vi "UHR-Fleezers Control (host) - 10.5.vi"() -> ()   [LabVIEW 2011]
uses:
  <vilib>/Utility/miscctls.llb/LVPoint32TypeDef.ctl
  <vilib>/Utility/miscctls.llb/LVMinMaxIncTypeDef.ctl
  <vilib>/userDefined/High Color/nirio_resource_hc.ctl
  <vilib>/Platform/TimedLoop/XDataNode/timing_clust.ctl
  <vilib>/Platform/TimedLoop/XDataNode/nitl_modes.ctl
  <vilib>/Platform/TimedLoop/XDataNode/wakeup.ctl
  <vilib>/vision/Avi1.llb/AviRefnum.ctl
  <vilib>/Instr/_visa.llb/VISA Configure Serial Port (Instr).vi
  <vilib>/FPGAPlugInAG/PCIe-7852R/niLvFpga_Open_PCIe-7852R.vi
  <vilib>/FPGAPlugInAG/PCIe-7852R/niLvFpga_Reset_PCIe-7852R.vi
  <vilib>/Utility/error.llb/Error Cluster From Error Code.vi
  <vilib>/rvi/errors/niLvFpgaAdjustHostInterfaceError.vi
  <vilib>/FPGAPlugInAG/PCIe-7852R/niLvFpga_Run_PCIe-7852R.vi
  <vilib>/express/express analysis/Spectral/Block/exnSpectralBlock spectral measurements PSD poly.vi
  <vilib>/express/express analysis/Spectral/Block/exnSpectralBlock spectral measurements PSD WFM.vi
  <vilib>/Waveform/WDTOps.llb/WDT Append Waveforms DBL.vi
  <vilib>/FPGAPlugInAG/PCIe-7852R/niLvFpga_Close_PCIe-7852R.vi
  openfpgaref.8.6.ctl
  <vilib>/Platform/TimedLoop/XDataNode/XDataNode.xnode
  <vilib>/rvi/interface/nirviOpenFPGA/nirviOpenFPGA.xnode
  FPGA Bitfiles/UHR-FleezersInst_FPGATarget_UHR-FleezersCont_AF27E570.lvbitx
  UHR-Fleezers Control (fpga) - 10.5.vi
  <vilib>/rvi/interface/nirviMethod/nirviMethod.xnode
  <vilib>/rvi/interface/nirviReadWriteControl/nirviReadWriteControl.xnode
  <vilib>/express/express analysis/Spectral/XNode/ExpressSpectralMeasurementsBlockNode.xnode
  <vilib>/rvi/interface/nirviCloseFPGA/nirviCloseFPGA.xnode
  <vilib>/Analysis/NI_AALBase.lvlib
  <vilib>/Platform/TimedLoop/XDataNode/XDNodeRunTimeDep.lvlib
  <vilib>/vision/NI_Vision_Development_Module.lvlib
  <vilib>/rvi/errors/niLvFpgaMergeErrorWithErrorCode.vi
  NiFpgaLv.dll
  <vilib>/FPGAPlugInAG/PCIe-7852R/niLvFpga_ConfigureFifo_PCIe-7852R.vi
  <vilib>/FPGAPlugInAG/PCIe-7852R/niLvFpga_ReadFifo_PCIe-7852R.vi
panel:
  out "Pump 3 cont disp":string="Left: ADig beads"
  out "Pump 1 cont disp":string="Right: DNA beads "
  in  "Ch 1 Inject Rate (ul/h)":dbl=25.0
  in  "Pump write delay (ms)":dbl=300.0
  in  "All Pump Parameters":T1={"Pump 1"={"Diameter (mm)"=4.61, "Units"=4.0, "Volume"=100.0, "Rate"=25.0}, "Pump 2"={"Diameter (mm)"=4.61, "Units"=3.0, "Volume"=0.0, "Rate"=0.0}, "Pump 3"={"Diameter (mm)"=4.61, "Units"=4.0, "Volume"=100.0, "Rate"=800.0}}
  in  "Ch 1 Inject Volume (uL)":dbl=100.0
  in  "Pump pause delay (ms)":u32
  in  "Ch 3 Inject Volume (uL)":dbl=100.0
  in  "Ch 3 Inject Rate (ul/h)":dbl=800.0
  in  "Flush Center Ch Volume (uL)":dbl=15.0
  in  "Flush Center Ch Rate (ul/m)":dbl=100.0
  in  "Inject Pump 2":bool caption="Inject Pump 2\n(Flush Center)"
  in  "Total Volume\nFlushed (uL)":dbl
  out "TTrig":cluster{dbl, dbl}(graph)
  in  "Sample Channel\nFlow":bool
  in  "Inject Pump 1":bool
  in  "Inject Pump 3":bool
  in  "Pump 1 contents":string="Bottom: DNA beads" caption="Contents"
  in  "Pump 3 contents":string="Top: ADig beads" caption="Contents"
  out "Time (s)":dbl=58.8
  in  "Index":dbl=1.0 caption="Save File Index" min=1.0 step=1.0
  in  "Scripts":T2(tab)
  in  "Fixed Traps Data\nScript":bool
  in  "Dump spot flow on?":bool=TRUE caption="Flow ON?"
  in  "Daq spot flow on":bool=TRUE caption="Flow ON?"
  in  "Cap 1 Samp Flow ON":bool=TRUE
  in  "Cap 2 Samp Flow ON":bool=TRUE
  in  "Got DNA bead":bool
  in  "Got ADig bead":bool
  in  "Cap 2 Flow ON":bool=TRUE
  in  "Cap 1 Flow ON":bool=TRUE
  in  "Cap 2 T ON":bool=TRUE
  in  "Move Cap. 2 (ADig Top)":bool
  in  "Move Cap. 1 (DNA Bottom)":bool
  in  "Cal/Data Acq. Spot":bool
  in  "Dump Beads":bool
  in  "Cap 1 T ON":bool=TRUE
  in  "Force FB Data\nScript":bool
  in  "Cap. 2 BD T1?\n(ADig T1, DNA T2)":bool
  in  "Offset 2 Set":dbl=2.0
  in  "Offset 1 Set":dbl
  in  "Cal @ (MHz)":dbl=15.25
  in  "W/ Offset 1":bool=TRUE
  in  "Offset 1 Start (MHz)":dbl=13.0
  in  "W/ Offset 2":bool
  in  "Offset 2 Start (MHz)":dbl=16.0
  in  "Cal Stage Position":i32=3
  in  "Flow ON during \nfishing?":bool=TRUE
  in  "Fish again after \nraster break?":bool=TRUE
  in  "Furthest Delta (MHz)":dbl=15.25 step=0.25
  in  "Green ON During Raster":bool
  in  "Move to Delta 2 (MHz)":dbl=13.0
  in  "Attempt Limit":dbl=15.0 caption="Limit"
  out "Attempts":dbl=15.0
  in  "Wait Before Save (s)":u32=1
  in  "Closest Delta (MHz)":dbl=9.25 step=0.25
  in  "Stop F (pN)":dbl=3.0
  in  "Then...":string(combo)="5"
  in  "Move to Delta 1 (MHz)":dbl=13.0
  in  "Tether Alarm?":bool=TRUE
  out "Tether":bool
  in  "TA Cancel Save?":bool
  in  "TA Green Off?":bool
  in  "Raster Set Upon Tether":u32=1
  in  "Save at end (5, 6)":bool
  in  "Start dipping after?":bool=TRUE
  in  "Green ON after FB ON?":bool
  in  "Remove Action Offset":bool
  in  "Stage Position To Establish FB":i32=3
  in  "Trap Trig Fl.":bool
  in  "Starting \nTrap Delta (MHz)":dbl=15.25
  in  "Trap Delta Before Moving":dbl=13.0
  in  "Wait (s)":u32=1
  in  "Green ON":bool
  in  "Start dipping after?":bool=TRUE
  in  "Fixed Traps Trap Delta (MHz)":dbl=15.25 caption="Trap Delta (MHz)"
  out "TTrig Fin Thresh (nm)":dbl
  out "TTrig Sig (nm)":dbl
  out "Threshold stored (nm)":dbl
  in  "Neg. TTrig FPGA":bool=TRUE
  in  "Test ttrig":bool
  in  "Trap Trig. (FPGA)":bool=TRUE
  out "Initializing":bool
  in  "Reinitialize":bool
  out "Triggered":bool
  out "Waiting":bool
  in  "Trap Trig. Fl.":bool
  in  "Wait to get offset (n)":u32=10
  in  "Threshold (nm)":dbl=15.0
  in  "Fl. ON time (n)":i32=90
  out "T1 x pos data":dbl[](array[numeric])=[-0.7109037245680824, -0.7109037245680824]
  out "max value":dbl=-0.9003514563721442
  out "min value":dbl=-1.184251119672945
  in  "Mean T1 Position\nto compare (nm)":dbl caption="Mean T1 for Comparison (nm)" format="%0.2f"
  out "mean":dbl=-1.0423012880225446 format="%0.2f"
  out "standard\ndeviation":dbl=0.2007473770965739 format="%0.2f"
  out "TTrig Sig (Int)":i64
  out "TTrig Fin Thresh (Int)":i64
  in  "FB Trig Integrate":u32=1
  in  "FB OFF when \nflow ON":bool
  in  "Flow ON \nduring return\nfrom dip?":bool=TRUE
  in  "Flow ON\nduring daq?":bool
  in  "Flow ON\nduring dip?":bool=TRUE
  in  "Cancel dwell":bool
  in  "Pause dwell \ntimer":bool
  in  "Dwell Duration (s)":i32=45
  in  "Green ON\nbefore dip?":bool
  in  "Cont. Repeat Dipping?":bool=TRUE
  in  "Dipping Delta (MHz)":dbl=15.0
  in  "Move trap \nbefore dip move?":bool
  in  "Save data\nafter return move?":bool
  in  "Green ON \nafter return?":bool=TRUE
  in  "Dip Trap Delta 2 (MHz)":dbl=15.0
  in  "Move trap \nafter return move?":bool
  in  "Dip Duration (s)":i32=15
  in  "Dip for Protein":bool
  in  "Dip Stage \nPosition":i32=5
  in  "Return Stage \nPosition":i32=3
  out "Dip Time (s)":i32=16
  out "Dip #":i32=5
  in  "Y change (mm)":dbl=3.0
  in  "Profile":bool
  out "Current Position":cluster{dbl, dbl, dbl}={1.5, -2.90746, -0.04434}
  in  "APD to Watch":bool
  out "Duration (s)":dbl
  in  "Action":string(combo)="Yank"
  in  "Fl. Triggered...":bool
  in  "Fl. Delta Thresh. (kHz)":dbl=0.6
  out "Waiting":bool
  out "Fl. High":bool
  in  "N pts to average":u16=6
  in  "Yank Delay (s)":dbl=3.5
  in  "Yank to Delta Array (MHz)":dbl[](array[numeric])=[16.3, 15.85, 14.85]
  in  "N Array El":u8=3 min=1 step=1
  in  "Random Choice":bool=TRUE
  in  "Force Yank":bool
  in  "Force Reset":bool
  in  "N Steps":dbl=20.0
  in  "Step Size (nm)":dbl=0.34
  in  "Save ave factor":dbl=1.0
  in  "Take Stepping Data":bool
  out "Sigma/Mean 2":dbl=0.36441577304438716 caption="Sigma/Mean" format="%#_2g"
  out "Rate sigma (Hz) 2":dbl=288.009932629414 caption="Sigma (Hz)" format="%0.2f"
  out "APD 2 Rate (Hz)":dbl=790.3333333333334 format="%#_3p"
  out "Primary Video Display":T3(plugin-control)
  out "Waveform Graph":dbl[](graph) caption="APD Line Scan"
  out "Messages":string="1:17 PM\tUHR-Fleezers ready.\r"
  in  "APD Ave N":dbl=10.0
  out "Int. Time (s)":dbl=3.0
  in  "Stop All":bool
  out "Sigma/Mean":dbl=0.18579745817752089 format="%#_2g"
  out "Rate sigma (Hz)":dbl=488.0899226323474 caption="Sigma (Hz)" format="%0.2f"
  in  "Tab Control 6":T4(tab)
  in  "APD 2 Offset":dbl
  in  "APD 1 Offset":dbl
  out "RMS (Ang)":dbl=6.074493407838442 format="%_2g"
  in  "Bead Sep. Int. Time (s)":dbl=3.0 caption="Int. Time (s)"
  in  "Below (kHz)":dbl=1.0
  in  "Above (kHz)":dbl=2.0
  in  "Adjust Scale\nto Mean":bool
  in  "Remove Offset":bool
  in  "Offset (nm)":dbl=-9.822711494362707 format="%#_3g"
  out "Mean":dbl=-2.4278133956623194 caption="Mean (pN)" format="%#_3g"
  out "Force":waveform(dbl)[](graph)=[{"t0"=timestamp(16.200000000000017 s since 1904-01-01), "dt"=0.15, "Y"=[-50.791733123427015, -51.19733990933295], "attributes"=variant("NI_ChannelName"=variant(string "T1 X"))}, {"t0"=timestamp(16.200000000000017 s since 1904-01-01), "dt"=0.15, "Y"=[45.92404992947972, 46.35376952063096], "attributes"=variant("NI_ChannelName"=variant(string "T2 X"))}]
  out "APD Chart":waveform(dbl)[](graph)=[{"t0"=timestamp(16.200000000000017 s since 1904-01-01), "dt"=0.15, "Y"=[2546.666666666667, 2813.3333333333335], "attributes"=variant("NI_ChannelName"=variant(string "APD 1"))}, {"t0"=timestamp(16.200000000000017 s since 1904-01-01), "dt"=0.15, "Y"=[720.0, 900.0], "attributes"=variant("NI_ChannelName"=variant(string "APD 2"))}]
  in  "Calibration":u16(ring)=2 items=["None", "Position", "Force"]
  out "T1 X":dbl=-50.99453651637998 caption="T1 X (pN)" format="%0.2f"
  out "T2 X":dbl=-46.13890972505534 caption="T2 X (pN)" format="%0.2f"
  out "Bead Separation":waveform(dbl)(graph)={"t0"=timestamp(16.200000000000017 s since 1904-01-01), "dt"=0.15, "Y"=[46.80967498827478, 46.86053516179577], "attributes"=variant("NI_ChannelName"=variant(string "T1 X"))}
  out "Bead Mean (nm)":dbl=47.53979851497442 caption="Mean (nm)" format="%0.2f"
  out "Difference":dbl=-97.13344624143532 caption="Difference (pN)" format="%.2g"
  in  "Take Detection Laser\nImage":bool
  out "APD 2":T3(plugin-control) caption="APD 2 (Cy5)"
  in  "Flip Green Filter":bool
  in  "Set X Only":bool
  in  "Set Y Only":bool
  out "APD 1":T3(plugin-control) caption="APD 1 (Cy3)"
  out "Detection Laser Y":T3(plugin-control)
  out "Pointer Y (V)":dbl=6.416201666310619 format="%_3g"
  out "Pointer X (V)":dbl=2.173967101046785 format="%_3g"
  in  "Set Confocal Spot (X-Y)":bool
  out "Detection Laser X":T3(plugin-control)
  out "Saved APD":dbl[][](graph)=[[2720.0, 2573.3333333333335, 2613.3333333333335, 2453.3333333333335, 2480.0, 2560.0, 2506.666666666667, 2466.666666666667, 2440.0, 2520.0, 2580.0, 2400.0, 2793.3333333333335, 2346.666666666667, 2853.3333333333335, 2453.3333333333335, 2513.3333333333335, 2713.3333333333335, 2720.0, 2633.3333333333335, 2560.0, 2693.3333333333335, 2620.0, 2613.3333333333335, 2453.3333333333335, 2566.666666666667, 2333.3333333333335, 2726.666666666667, 2806.666666666667, 2526.666666666667, 2640.0, 2606.666666666667, 2680.0, 2793.3333333333335, 2546.666666666667, 2473.3333333333335, 2593.3333333333335, 2653.3333333333335, 2566.666666666667, 2493.3333333333335, 2766.666666666667, 2446.666666666667, 2466.666666666667, 2746.666666666667, 2800.0, 2306.666666666667, 2426.666666666667, 2593.3333333333335, 2633.3333333333335, 2326.666666666667, 2693.3333333333335, 2680.0, 2726.666666666667, 2546.666666666667, 2573.3333333333335, 2446.666666666667, 2513.3333333333335, 2606.666666666667, 2686.666666666667, 2460.0, 2653.3333333333335, 2660.0, 2406.666666666667, 2706.666666666667, 2520.0, 2420.0, 2560.0, 2553.3333333333335, 2566.666666666667, 2406.666666666667, 2546.666666666667, 2433.3333333333335, 2446.666666666667, 2480.0, 2520.0, 2593.3333333333335, 2653.3333333333335, 2580.0, 2600.0, 2626.666666666667, 2686.666666666667, 2593.3333333333335, 2540.0, 2580.0, 2586.666666666667, 2626.666666666667, 2426.666666666667, 2800.0, 2693.3333333333335, 2666.666666666667, 2553.3333333333335, 2746.666666666667, 2693.3333333333335, 2880.0, 2480.0, 2540.0, 2613.3333333333335, 2573.3333333333335, 2746.666666666667, 2633.3333333333335, 3006.666666666667, 2880.0, 2813.3333333333335, 2660.0, 2653.3333333333335, 2513.3333333333335, 2526.666666666667, 2800.0, 2673.3333333333335, 2286.666666666667, 2593.3333333333335, 2260.0, 2620.0, 2653.3333333333335, 2753.3333333333335, 2413.3333333333335, 2433.3333333333335, 2506.666666666667, 2340.0, 2800.0, 2653.3333333333335, 2473.3333333333335, 2320.0, 2600.0, 2613.3333333333335, 2613.3333333333335, 2546.666666666667, 2586.666666666667, 2506.666666666667, 2860.0, 2273.3333333333335, 2540.0, 2486.666666666667, 2493.3333333333335, 2626.666666666667, 2620.0, 2466.666666666667, 2600.0, 2840.0, 2746.666666666667, 2580.0, 2760.0, 2686.666666666667, 2446.666666666667, 2600.0, 2533.3333333333335, 2800.0, 2933.3333333333335, 2580.0, 2400.0, 2540.0, 2600.0, 2580.0, 2360.0, 2480.0, 2580.0, 2486.666666666667, 2520.0, 2546.666666666667, 2626.666666666667, 2400.0, 2740.0, 2573.3333333333335, 2413.3333333333335, 2566.666666666667, 2633.3333333333335, 2500.0, 2680.0, 2393.3333333333335, 2533.3333333333335, 2633.3333333333335, 2406.666666666667, 2600.0, 2566.666666666667, 2860.0, 2713.3333333333335, 2506.666666666667, 2726.666666666667, 2560.0, 2693.3333333333335, 2633.3333333333335, 2473.3333333333335, 2593.3333333333335, 2533.3333333333335, 2533.3333333333335, 2753.3333333333335, 2440.0, 2680.0, 2593.3333333333335, 2560.0, 2440.0, 2460.0, 2506.666666666667, 2593.3333333333335, 2613.3333333333335, 2433.3333333333335, 2706.666666666667, 2666.666666666667, 2533.3333333333335, 2593.3333333333335, 2686.666666666667, 2320.0, 2553.3333333333335, 2853.3333333333335, 2686.666666666667, 2620.0, 2673.3333333333335, 2493.3333333333335, 2333.3333333333335, 2593.3333333333335, 2546.666666666667, 2553.3333333333335, 2706.666666666667, 2613.3333333333335, 2466.666666666667, 2433.3333333333335, 2633.3333333333335, 2920.0, 2480.0, 2580.0, 2346.666666666667, 2613.3333333333335, 2566.666666666667, 2626.666666666667, 2453.3333333333335, 2586.666666666667, 2700.0, 2420.0, 2520.0, 2573.3333333333335, 2626.666666666667, 2673.3333333333335, 2446.666666666667, 2526.666666666667, 2506.666666666667, 2640.0, 2500.0, 2500.0, 2473.3333333333335, 2640.0, 2500.0, 2373.3333333333335, 2706.666666666667, 2666.666666666667, 2853.3333333333335, 2460.0, 2533.3333333333335, 2706.666666666667, 2526.666666666667, 2760.0, 2506.666666666667, 2566.666666666667, 2653.3333333333335, 2646.666666666667, 2873.3333333333335, 2613.3333333333335, 2493.3333333333335, 2513.3333333333335, 2640.0, 2486.666666666667, 2740.0, 2660.0, 2653.3333333333335, 2633.3333333333335, 2906.666666666667, 2860.0, 2653.3333333333335, 2633.3333333333335, 2640.0, 2406.666666666667, 2540.0, 2613.3333333333335, 2393.3333333333335, 2506.666666666667, 2600.0, 2546.666666666667, 2653.3333333333335, 2513.3333333333335, 2633.3333333333335, 2386.666666666667, 2546.666666666667, 2893.3333333333335, 2733.3333333333335, 2593.3333333333335, 2573.3333333333335, 2580.0, 2653.3333333333335, 2666.666666666667, 2680.0, 2580.0, 2393.3333333333335, 2780.0, 2413.3333333333335, 2606.666666666667, 2600.0, 2540.0, 2546.666666666667, 2833.3333333333335, 2513.3333333333335, 2573.3333333333335, 2693.3333333333335, 2840.0, 2580.0, 2700.0, 2793.3333333333335, 2546.666666666667, 2606.666666666667, 2453.3333333333335, 2593.3333333333335, 2500.0, 2520.0, 2640.0, 2813.3333333333335, 2813.3333333333335, 2493.3333333333335, 2686.666666666667, 2673.3333333333335, 2533.3333333333335, 2480.0, 2606.666666666667, 2680.0, 2646.666666666667, 2646.666666666667, 2626.666666666667, 2433.3333333333335, 2633.3333333333335, 2540.0, 2506.666666666667, 2620.0, 2553.3333333333335, 2480.0, 2533.3333333333335, 2620.0, 2860.0, 2506.666666666667, 2753.3333333333335, 2400.0, 2493.3333333333335, 2513.3333333333335, 2713.3333333333335, 2673.3333333333335, 2473.3333333333335, 2720.0, 2580.0, 2613.3333333333335, 2533.3333333333335, 2680.0, 2413.3333333333335, 2373.3333333333335, 2566.666666666667, 2560.0, 2806.666666666667, 2633.3333333333335, 2520.0, 2526.666666666667, 2633.3333333333335, 2753.3333333333335, 2746.666666666667, 2780.0, 2780.0, 2466.666666666667, 2573.3333333333335, 2600.0, 2706.666666666667, 2506.666666666667, 2500.0, 2586.666666666667, 2646.666666666667, 2620.0, 2400.0, 2726.666666666667, 2666.666666666667, 2606.666666666667, 2553.3333333333335, 2726.666666666667, 2720.0, 2546.666666666667, 2606.666666666667, 2506.666666666667, 2573.3333333333335, 2593.3333333333335, 2660.0, 2600.0, 2580.0, 2440.0, 2846.666666666667, 2406.666666666667, 2600.0, 2573.3333333333335, 2533.3333333333335], [766.6666666666667, 786.6666666666667, 813.3333333333334, 806.6666666666667, 813.3333333333334, 813.3333333333334, 813.3333333333334, 760.0, 846.6666666666667, 873.3333333333334, 853.3333333333334, 813.3333333333334, 880.0, 853.3333333333334, 813.3333333333334, 713.3333333333334, 820.0, 826.6666666666667, 846.6666666666667, 760.0, 833.3333333333334, 733.3333333333334, 800.0, 786.6666666666667, 766.6666666666667, 760.0, 740.0, 733.3333333333334, 840.0, 773.3333333333334, 800.0, 846.6666666666667, 853.3333333333334, 913.3333333333334, 733.3333333333334, 793.3333333333334, 773.3333333333334, 793.3333333333334, 853.3333333333334, 800.0, 833.3333333333334, 893.3333333333334, 886.6666666666667, 766.6666666666667, 706.6666666666667, 813.3333333333334, 733.3333333333334, 780.0, 593.3333333333334, 846.6666666666667, 720.0, 740.0, 800.0, 726.6666666666667, 833.3333333333334, 800.0, 846.6666666666667, 740.0, 726.6666666666667, 780.0, 733.3333333333334, 706.6666666666667, 740.0, 806.6666666666667, 666.6666666666667, 980.0, 873.3333333333334, 933.3333333333334, 793.3333333333334, 913.3333333333334, 780.0, 786.6666666666667, 746.6666666666667, 846.6666666666667, 726.6666666666667, 786.6666666666667, 786.6666666666667, 686.6666666666667, 820.0, 746.6666666666667, 846.6666666666667, 720.0, 733.3333333333334, 800.0, 706.6666666666667, 766.6666666666667, 773.3333333333334, 780.0, 833.3333333333334, 853.3333333333334, 733.3333333333334, 820.0, 706.6666666666667, 673.3333333333334, 833.3333333333334, 806.6666666666667, 813.3333333333334, 700.0, 806.6666666666667, 793.3333333333334, 753.3333333333334, 886.6666666666667, 746.6666666666667, 820.0, 693.3333333333334, 720.0, 786.6666666666667, 920.0, 893.3333333333334, 760.0, 840.0, 713.3333333333334, 846.6666666666667, 793.3333333333334, 793.3333333333334, 773.3333333333334, 786.6666666666667, 813.3333333333334, 926.6666666666667, 806.6666666666667, 786.6666666666667, 820.0, 800.0, 733.3333333333334, 813.3333333333334, 826.6666666666667, 846.6666666666667, 720.0, 773.3333333333334, 760.0, 873.3333333333334, 866.6666666666667, 880.0, 766.6666666666667, 746.6666666666667, 720.0, 893.3333333333334, 793.3333333333334, 813.3333333333334, 900.0, 746.6666666666667, 866.6666666666667, 833.3333333333334, 780.0, 833.3333333333334, 733.3333333333334, 733.3333333333334, 613.3333333333334, 806.6666666666667, 880.0, 853.3333333333334, 753.3333333333334, 746.6666666666667, 893.3333333333334, 800.0, 873.3333333333334, 933.3333333333334, 733.3333333333334, 693.3333333333334, 920.0, 993.3333333333334, 720.0, 853.3333333333334, 706.6666666666667, 686.6666666666667, 793.3333333333334, 726.6666666666667, 806.6666666666667, 860.0, 813.3333333333334, 806.6666666666667, 666.6666666666667, 860.0, 793.3333333333334, 800.0, 773.3333333333334, 653.3333333333334, 853.3333333333334, 720.0, 806.6666666666667, 640.0, 993.3333333333334, 773.3333333333334, 833.3333333333334, 673.3333333333334, 786.6666666666667, 780.0, 846.6666666666667, 786.6666666666667, 866.6666666666667, 813.3333333333334, 893.3333333333334, 813.3333333333334, 746.6666666666667, 806.6666666666667, 900.0, 740.0, 813.3333333333334, 973.3333333333334, 873.3333333333334, 780.0, 720.0, 860.0, 833.3333333333334, 633.3333333333334, 746.6666666666667, 813.3333333333334, 653.3333333333334, 813.3333333333334, 940.0, 973.3333333333334, 853.3333333333334, 820.0, 773.3333333333334, 760.0, 860.0, 860.0, 733.3333333333334, 760.0, 940.0, 713.3333333333334, 713.3333333333334, 913.3333333333334, 926.6666666666667, 840.0, 766.6666666666667, 840.0, 853.3333333333334, 753.3333333333334, 746.6666666666667, 733.3333333333334, 760.0, 793.3333333333334, 780.0, 860.0, 740.0, 840.0, 853.3333333333334, 760.0, 820.0, 926.6666666666667, 566.6666666666667, 820.0, 820.0, 846.6666666666667, 846.6666666666667, 960.0, 773.3333333333334, 866.6666666666667, 746.6666666666667, 813.3333333333334, 973.3333333333334, 866.6666666666667, 686.6666666666667, 826.6666666666667, 853.3333333333334, 906.6666666666667, 866.6666666666667, 706.6666666666667, 813.3333333333334, 786.6666666666667, 800.0, 806.6666666666667, 813.3333333333334, 693.3333333333334, 886.6666666666667, 760.0, 953.3333333333334, 720.0, 873.3333333333334, 826.6666666666667, 866.6666666666667, 786.6666666666667, 733.3333333333334, 873.3333333333334, 720.0, 813.3333333333334, 780.0, 753.3333333333334, 673.3333333333334, 760.0, 833.3333333333334, 700.0, 853.3333333333334, 773.3333333333334, 926.6666666666667, 900.0, 753.3333333333334, 886.6666666666667, 820.0, 820.0, 713.3333333333334, 813.3333333333334, 720.0, 840.0, 880.0, 880.0, 773.3333333333334, 746.6666666666667, 800.0, 920.0, 900.0, 766.6666666666667, 773.3333333333334, 766.6666666666667, 800.0, 860.0, 893.3333333333334, 680.0, 780.0, 760.0, 713.3333333333334, 660.0, 806.6666666666667, 920.0, 686.6666666666667, 806.6666666666667, 793.3333333333334, 773.3333333333334, 753.3333333333334, 873.3333333333334, 753.3333333333334, 860.0, 826.6666666666667, 793.3333333333334, 833.3333333333334, 773.3333333333334, 906.6666666666667, 766.6666666666667, 813.3333333333334, 766.6666666666667, 846.6666666666667, 673.3333333333334, 826.6666666666667, 826.6666666666667, 746.6666666666667, 746.6666666666667, 873.3333333333334, 786.6666666666667, 700.0, 893.3333333333334, 786.6666666666667, 913.3333333333334, 820.0, 833.3333333333334, 820.0, 893.3333333333334, 826.6666666666667, 746.6666666666667, 760.0, 753.3333333333334, 746.6666666666667, 746.6666666666667, 893.3333333333334, 753.3333333333334, 833.3333333333334, 826.6666666666667, 880.0, 813.3333333333334, 880.0, 666.6666666666667, 806.6666666666667, 773.3333333333334, 913.3333333333334, 726.6666666666667, 793.3333333333334, 880.0, 840.0, 833.3333333333334, 866.6666666666667, 946.6666666666667, 813.3333333333334, 846.6666666666667, 826.6666666666667, 813.3333333333334, 766.6666666666667, 766.6666666666667, 720.0, 746.6666666666667, 786.6666666666667, 820.0, 846.6666666666667, 853.3333333333334, 786.6666666666667, 800.0, 820.0, 746.6666666666667, 720.0, 840.0, 806.6666666666667]] caption="Most Recent Time Trace"
  out "Trap Delta Graph":dbl[](graph)=[47.20544674943777, 46.38357473836321, 45.83818091067762, 46.35063870780333, 46.57328126817542, 46.26983509094593, 46.207785466693664, 46.12090860203374, 46.75480485600748, 45.89837089817051, 46.52249402855391, 46.74710833092389, 46.48685302300156, 45.980928940659666, 46.08378499907887, 46.29776150204533, 46.52270355958599, 45.13312371565935, 45.45279739842816, 46.12725237006576, 45.934373783395515, 46.11062060160292, 45.819898737241985, 46.427428605258385, 46.4251508638754, 46.259210180234035, 46.536328123957716, 45.71916638273997, 46.53364731772011, 46.193012961034, 46.75119956112418, 46.541703884601716, 46.49256378963746, 46.28722689614035, 47.06115445826505, 46.93267094186844, 46.00494603544506, 46.76063596928016, 46.342510510696414, 46.45985325566586, 46.38609146330846, 46.56011036664573, 46.78009201374856, 46.06330853754797, 45.511271587741035, 45.34662244853736, 46.17450546200233, 46.20649996594419, 46.37474271434699, 46.026748302381534, 45.5567280877173, 45.99975938911392, 44.660215879237214, 45.8487237846431, 46.104322288890685, 46.948445853152506, 46.59561462300782, 46.195067267325655, 45.61273562855426, 46.35745428628489, 46.37827046492161, 46.310155347688934, 46.2829444903622, 46.3597756481595, 45.541201308487345, 46.69975389865577, 46.471358477380804, 46.92663001022483, 46.58686909319992, 46.37677654594965, 46.59541766001048, 46.7910410011245, 45.98027034700526, 46.19745620593365, 45.970726941628655, 46.937427032893865, 46.61827065262689, 47.492195371928304, 46.609536802213015, 46.467451731931575, 46.43332804681613, 46.39826316003827, 47.41675721906755, 46.44034533370349, 46.71929038633529, 46.06840779135548, 46.86518149702191, 47.20756883644232, 46.82935338918453, 46.90743803093055, 45.51252051538394, 47.24326673407994, 47.72875647707973, 46.72602030048229, 47.384475140534036, 47.30082048895572, 48.07845904973122, 46.423143708556, 46.496401779930736, 46.66161761723579, 46.364686383535755, 46.84723627239062, 46.494614135825955, 46.2750025397515, 46.23198085606502, 46.375794104870906, 46.13019512162806, 46.71238392521188, 46.51013892816643, 47.089569197134566, 46.35511433767981, 46.34759345874086, 46.25067399284127, 46.98462017803094, 47.02395331921302, 46.65155678882006, 46.321890322751685, 45.6835009219064, 45.87994019887792, 46.8658480783014, 46.44286319640274, 46.262471040955475, 46.914186422887, 45.92051455412998, 47.413190381915044, 46.31570035057068, 45.901473731967414, 47.3973466321129, 46.559605367656545, 47.44788671547947, 47.06091656936151, 46.407753131563865, 45.79400378596769, 46.36440775731673, 46.20021291782611, 46.626803855129296, 46.57989326818925, 46.93019099456963, 46.405901234598176, 47.47024503240657, 46.94501321909864, 47.433305792174096, 46.57314592783875, 45.77155448986561, 46.85135093280839, 46.34374951571358, 45.90860353770337, 46.76809212254916, 46.791019801339885, 45.94328559525884, 46.51508389774152, 46.417402677528955, 46.22370593813751, 47.061806653544565, 45.848808906630595, 46.619660064521966, 46.657935496503754, 45.99001486688685, 46.52004794686245, 47.66084894068457, 46.23016320716654, 47.0223240362463, 46.36738118514596, 46.8010129768857, 46.91598786111915, 46.943159583517215, 46.32543069125178, 46.550212551764034, 45.58512269658003, 46.69156580484993, 46.43476329001264, 45.834629618577466, 46.1140698840063, 47.28192166795104, 46.6080172766989, 46.81243435411666, 46.35949247601495, 47.023358994777126, 46.95847383066577, 46.514425539119244, 46.298839114129336, 46.88552371438767, 46.28134853208782, 46.86832706415841, 46.049964609114184, 46.06997314928573, 46.3585212932271, 46.40886017981835, 45.9794448155141, 46.06734037951817, 46.01190511000904, 47.08901062982436, 45.65151203581401, 45.49765396093453, 45.58613471941008, 45.931848042336796, 46.09606020305493, 46.79726278098475, 45.53133688464315, 46.856940025409116, 46.5092293835677, 46.18284415269427, 46.13054289742972, 45.97260177637533, 46.006373431335064, 46.04988123169922, 46.01074170138004, 46.90224306777496, 46.3227898619963, 47.103533536483766, 47.21133615073923, 46.8913680055975, 46.62682837519351, 47.53713685608041, 46.13778467041497, 46.6692751114917, 47.11340861422174, 45.81362704226548, 46.02226189955444, 46.70098430809374, 46.9272368792039, 46.70584815983797, 47.518318240250935, 47.31316945209845, 46.27084532868322, 46.905472631555185, 47.323881893679086, 46.42931996166523, 46.62825802471117, 46.36537141579139, 47.221612368324756, 46.89327030819767, 47.68470857707025, 45.59050231121266, 46.43044939438197, 46.44540550367991, 47.1087157758589, 46.930637317511255, 45.75274812282625, 46.90769159391856, 46.98508896949595, 46.423609890313756, 47.13682341908965, 48.20536165960549, 47.15235560328587, 46.29894064132209, 47.64085705084754, 46.61439161657212, 47.229688263465746, 47.25379338518748, 46.61793600921523, 47.64346472854267, 47.60230865364845, 47.46595880879771, 47.00342389717902, 46.50642406509242, 47.073063990431635, 46.4132534425532, 47.15340819100241, 47.0151201253728, 46.23248972350332, 47.02335187697453, 46.756645425712165, 47.21844463782004, 46.82960077469973, 46.20181266495983, 46.677945311108985, 46.28453548537094, 47.010554930333015, 47.23557630480015, 46.049685708844905, 46.75631760649465, 46.911369657048894, 46.90400035310837, 47.47010123253169, 47.5335605651366, 46.19298683353831, 47.42084272116337, 46.440405076321085, 46.93603760368411, 47.52609037430203, 47.29013874104926, 47.74247780867337, 46.28264100099007, 46.23620039145909, 47.91838298167288, 46.27934280296891, 46.91324856208148, 46.46364902172071, 46.736791894666865, 47.39736180824839, 47.43734774233009, 46.81632250451027, 46.39751547983495, 47.61933911260256, 46.52309972554512, 48.079390490959426, 46.84754638483891, 46.95443858157536, 46.206737938217074, 46.800741751995574, 46.631363788227745, 47.42119039647993, 47.66160150830102, 45.252514693674684, 47.05278767055073, 45.99755200462256, 47.783120488885416, 46.55265606790981, 47.02960054153924, 46.935163090335564, 47.164591634852385, 47.24998564712884, 46.24634878151507, 46.716326655370054, 46.775230695912214, 46.3169357701063, 46.823617566670364, 46.21599600948743, 46.44735929375254, 45.80517711687666, 46.92185700699697, 46.411098455925426, 45.610887449466006, 46.953781294180075, 46.24342708094828, 46.987282791833294, 45.92203712498723, 45.96938932373995, 45.76818907239645, 46.101899185827776, 46.32801468270638, 46.97575649835112, 47.3566885577316, 46.6358364849079, 46.48481821111396, 47.12286691063504, 46.99408092691276, 47.30388936102982, 46.98293422235808, 47.42503603670339, 48.157962325575525, 46.09681071786015, 46.73221531409324, 47.219889646569484, 47.193109471306045, 47.45450663820476, 45.9114309476975, 46.75474687829713, 47.25931435523499, 46.74989361548667, 45.95352713387466, 47.287517700891456, 46.93716275892102, 46.56970348221158, 47.24147620230134, 46.57691994038676, 47.93347914826508, 46.56263102063862, 47.46290028361791, 46.77173029309408, 47.167558888427706, 47.10359440174476, 47.58936198782784, 47.69255940370404, 46.75703783278429, 46.432325237845376, 46.06155923680335, 46.032815699171564, 46.110376712450474, 47.48062736221716, 46.64664467730417, 46.57373381096677, 45.87891279189138, 46.94561843630895, 46.58655399454905, 47.33721637710819, 46.782102762982575, 47.25023779816355, 46.36149144860575, 47.00942768082545, 46.04829311591557, 46.518913411484206, 46.47685531631707, 46.30976158613113, 46.86945955204946, 46.4456839198575, 46.32942914270565, 46.05887349576837, 46.74406170178314] caption="Most Recent Time Trace"
  out "Save APD Deriv":dbl[][](graph)=[[0.0, 0.0, 0.0, -53.333333333333485, -71.11111111111131, -81.11111111111131, 0.0, 75.55555555555566, 126.66666666666697, 134.44444444444434, 67.77777777777783, 27.777777777777374, -63.333333333333485, -86.66666666666652, -71.11111111111086, 22.222222222222626, 123.33333333333303, 54.44444444444434, 16.666666666666515, -121.11111111111086, -36.666666666666515, -42.22222222222217, 34.44444444444434, -30.0, -66.66666666666652, -30.0, 44.44444444444434, 96.66666666666652, 10.0, -53.333333333333485, -14.444444444444343, 26.666666666666515, 13.333333333333485, -68.88888888888914, -91.11111111111131, -50.0, -47.77777777777783, -1.1111111111108585, 34.44444444444434, 115.55555555555566, 120.0, 58.88888888888869, 6.66666666666697, -30.0, 28.88888888888914, 45.5555555555552, 112.22222222222217, 15.555555555555657, -17.77777777777783, -107.77777777777783, 93.33333333333348, 160.0, 156.66666666666652, -81.11111111111131, -214.44444444444434, -231.11111111111086, -146.66666666666697, -26.666666666666515, 40.0, 26.66666666666697, -14.444444444444798, -32.22222222222217, 4.444444444444343, 12.222222222222626, 90.0, 6.66666666666697, -20.0, -114.44444444444434, -3.333333333333485, 123.33333333333303, 158.8888888888887, 127.77777777777783, -48.88888888888869, 1.1111111111113132, -35.55555555555566, 41.11111111111086, -156.66666666666697, -117.77777777777783, -141.11111111111086, 30.0, 30.0, 48.88888888888869, 14.444444444444343, 7.777777777777828, 1.1111111111113132, -30.0, -38.88888888888869, 78.88888888888869, 137.77777777777828, 154.44444444444434, -31.11111111111086, -81.11111111111131, -90.0, -10.0, 12.222222222222172, -57.77777777777828, -63.333333333333485, -85.55555555555566, 57.77777777777828, 65.55555555555566, 76.66666666666697, 3.33333333333303, 28.888888888888687, 62.22222222222217, -23.33333333333303, -87.77777777777737, -88.88888888888914, -13.333333333333485, 96.66666666666652, 27.77777777777783, 42.22222222222217, -93.33333333333348, -53.33333333333303, -36.666666666666515, 6.666666666666515, 53.33333333333303, 2.2222222222221717, 27.77777777777783, -65.55555555555566, -17.77777777777783, -72.22222222222217, 40.0, 50.0, 156.66666666666697, 80.0, 6.666666666666515, -44.4444444444448, 3.333333333333485, 32.222222222222626, -6.666666666666515, -54.44444444444434, 3.33333333333303, 138.8888888888887, 134.44444444444434, 47.77777777777783, -161.11111111111086, -206.66666666666652, -150.0, -45.55555555555566, 38.88888888888869, 71.11111111111131, 95.55555555555566, 97.77777777777783, 28.888888888888687, -8.888888888889142, -27.77777777777783, -57.77777777777783, -66.66666666666652, -35.55555555555566, 25.555555555555657, 111.11111111111131, 60.0, 91.11111111111086, -53.333333333333485, -67.77777777777737, -140.0, 33.333333333333485, 78.88888888888869, 116.66666666666697, -67.77777777777783, -57.77777777777783, -54.44444444444434, 32.22222222222217, -38.88888888888869, -66.66666666666697, -72.22222222222217, 46.666666666666515, 77.77777777777783, 66.66666666666652, -47.77777777777783, -81.11111111111131, 6.666666666666515, 35.55555555555566, 45.55555555555566, -82.22222222222217, -32.22222222222217, -13.33333333333303, 83.33333333333348, 68.88888888888869, 126.66666666666652, 70.0, 15.555555555555657, -144.44444444444434, -92.22222222222217, -107.77777777777783, 48.88888888888869, 4.444444444444343, 123.33333333333348, 18.88888888888914, 17.77777777777783, -85.55555555555566, -41.11111111111131, 6.666666666666515, -2.2222222222221717, -18.888888888888687], [0.0, 0.0, 0.0, 3.3333333333333712, 20.0, 26.666666666666742, 50.0, 1.1111111111110858, -8.888888888888914, -56.66666666666663, -17.777777777777715, -24.444444444444457, -16.666666666666742, -38.888888888888914, -24.444444444444457, 8.888888888888914, 73.33333333333337, 54.44444444444446, 21.111111111111086, -46.66666666666674, 1.1111111111110858, 28.888888888888914, 25.555555555555657, -43.33333333333326, -93.33333333333326, -81.1111111111112, -43.33333333333337, 24.444444444444343, 55.55555555555554, 50.0, -14.444444444444343, -42.22222222222217, -15.555555555555543, 77.77777777777771, 111.11111111111109, 74.44444444444446, -22.22222222222217, -81.11111111111109, -83.33333333333337, -52.222222222222285, -11.111111111111086, 14.444444444444457, 3.3333333333333712, -7.777777777777828, 7.777777777777828, 36.66666666666663, 10.0, -23.33333333333337, -43.33333333333326, 22.222222222222285, 30.0, 45.55555555555554, -22.222222222222285, -11.1111111111112, -5.555555555555657, 48.888888888888914, 26.666666666666742, -2.2222222222221717, -17.777777777777715, 8.888888888888914, 30.0, 11.111111111111086, -20.0, -33.33333333333337, -22.222222222222285, 10.0, 30.0, 18.888888888888914, -6.6666666666667425, -8.888888888888914, 26.666666666666742, 23.33333333333337, -12.222222222222172, -81.1111111111112, -56.66666666666663, -25.555555555555543, 67.77777777777783, 53.33333333333326, 56.66666666666663, 3.3333333333332575, 12.222222222222285, -15.555555555555543, -33.33333333333326, -70.0, -33.33333333333326, -12.222222222222285, 37.777777777777715, 2.2222222222221717, 8.888888888888914, -32.22222222222217, -5.555555555555543, 5.555555555555543, 15.555555555555543, 4.444444444444457, -4.444444444444457, 47.77777777777783, 37.777777777777715, 38.888888888888914, -27.77777777777783, 31.111111111111086, -12.222222222222172, 36.66666666666663, -88.8888888888888, -60.0, -73.33333333333326, 78.8888888888888, 105.55555555555554, 73.33333333333326, -40.0, -43.33333333333337, -53.33333333333326, 26.666666666666742, -6.666666666666629, 70.0, -27.77777777777783, -31.1111111111112, -95.55555555555566, -22.22222222222217, 30.0, 51.111111111111086, 16.66666666666663, -25.555555555555543, -7.777777777777715, 50.0, 54.44444444444446, 51.1111111111112, -18.8888888888888, -3.3333333333332575, -21.111111111111086, 3.3333333333332575, -23.33333333333337, -46.66666666666674, -31.111111111111086, 5.555555555555543, 26.66666666666663, 35.55555555555554, -17.777777777777715, -13.333333333333258, -48.888888888888914, -32.222222222222285, -32.222222222222285, -22.22222222222217, 38.888888888888914, 48.888888888888914, 81.11111111111109, 7.777777777777715, -22.222222222222285, -45.55555555555554, 2.2222222222222854, 24.444444444444457, 38.888888888888914, 0.0, 1.1111111111110858, -26.666666666666742, -21.111111111111086, -40.0, -76.66666666666663, -38.888888888888914, -2.2222222222221717, 55.55555555555554, 34.44444444444446, 27.77777777777783, 34.44444444444446, 40.0, 7.777777777777715, -11.111111111111086, -50.0, -33.33333333333326, -30.0, -2.2222222222222854, 16.66666666666663, 34.44444444444446, 64.44444444444446, 53.33333333333326, -3.3333333333333712, -56.66666666666663, -76.66666666666663, -25.555555555555543, 34.44444444444446, 56.66666666666663, 24.444444444444457, -13.333333333333371, -51.111111111111086, 8.8888888888888, 14.444444444444457, 83.33333333333337, 34.44444444444457, 12.222222222222285, -73.33333333333337, -88.88888888888891, -54.44444444444446, 16.666666666666742, 54.44444444444434, 6.666666666666629, -17.77777777777783]] caption="Most Recent Time Trace"
  out "Delta Fl. 1":dbl=-18.888888888888687
  out "Delta Fl. 2":dbl=-17.77777777777783
  out "All Signals":waveform(dbl)[](graph)=[{"t0"=timestamp(16.200000000000017 s since 1904-01-01), "dt"=0.15, "Y"=[3820.0, 4220.0], "attributes"=variant("NI_ChannelName"=variant(string "APD 1"))}, {"t0"=timestamp(16.200000000000017 s since 1904-01-01), "dt"=0.15, "Y"=[1080.0, 1350.0], "attributes"=variant("NI_ChannelName"=variant(string "APD 2"))}, {"t0"=timestamp(16.200000000000017 s since 1904-01-01), "dt"=0.15, "Y"=[-0.5988837991219723, -0.6005281703716233], "attributes"=variant("NI_ChannelName"=variant(string "T1 Y"))}, {"t0"=timestamp(16.200000000000017 s since 1904-01-01), "dt"=0.15, "Y"=[-0.1906275283822458, -0.19289872792319143], "attributes"=variant("NI_ChannelName"=variant(string "T1 X"))}, {"t0"=timestamp(16.200000000000017 s since 1904-01-01), "dt"=0.15, "Y"=[0.007211951048310644, 0.007210547196874748], "attributes"=variant("NI_ChannelName"=variant(string "T1 Sum"))}, {"t0"=timestamp(16.200000000000017 s since 1904-01-01), "dt"=0.15, "Y"=[-0.6088199063971451, -0.6110046413795541], "attributes"=variant("NI_ChannelName"=variant(string "T2 Y"))}, {"t0"=timestamp(16.200000000000017 s since 1904-01-01), "dt"=0.15, "Y"=[-0.20076800461133065, -0.20344643613150135], "attributes"=variant("NI_ChannelName"=variant(string "T2 X"))}, {"t0"=timestamp(16.200000000000017 s since 1904-01-01), "dt"=0.15, "Y"=[0.007201666310617233, 0.0071991332743307265], "attributes"=variant("NI_ChannelName"=variant(string "T2 Sum"))}, {"t0"=timestamp(16.200000000000017 s since 1904-01-01), "dt"=0.15, "Y"=[-0.011619833765516605, -0.014270969510904575], "attributes"=variant("NI_ChannelName"=variant(string "T1 FB X"))}, {"t0"=timestamp(16.200000000000017 s since 1904-01-01), "dt"=0.15, "Y"=[0.008562486648151986, 0.008559129612109627], "attributes"=variant("NI_ChannelName"=variant(string "T1 FB Sum"))}, {"t0"=timestamp(16.200000000000017 s since 1904-01-01), "dt"=0.15, "Y"=[-0.01973675035686103, -0.02249976801848294], "attributes"=variant("NI_ChannelName"=variant(string "T2 FB X"))}, {"t0"=timestamp(16.200000000000017 s since 1904-01-01), "dt"=0.15, "Y"=[0.008505020294808686, 0.008491073335978157], "attributes"=variant("NI_ChannelName"=variant(string "T2 FB Sum"))}, {"t0"=timestamp(16.200000000000017 s since 1904-01-01), "dt"=0.15, "Y"=[-4.009360785519027, -4.01544459589373], "attributes"=variant("NI_ChannelName"=variant(string "PSD Y"))}, {"t0"=timestamp(16.200000000000017 s since 1904-01-01), "dt"=0.15, "Y"=[-0.2765283989137259, -0.2775512713088634], "attributes"=variant("NI_ChannelName"=variant(string "PSD X"))}, {"t0"=timestamp(16.200000000000017 s since 1904-01-01), "dt"=0.15, "Y"=[-0.024687459944455828, -0.024652394177067907], "attributes"=variant("NI_ChannelName"=variant(string "PSD Y Sum"))}]
  in  "Signals to Plot":i32(listbox)
  out "Trap Disp. Freq. (Hz)":dbl=6.666666666666667 caption="Freq. (Hz)" format="%#_6p"
  out "Display Period (s)":dbl=0.15 caption="Period (s)" format="%#_6p"
  in  "Trap Disp. Downsample":dbl=10000.0 caption="Downsample" max=20000.0
  in  "APD Disp. Scale":dbl=0.1 caption="Scale (Divide,\nfor above plot only)"
  in  "APD Disp. Downsample":dbl=15.0 caption="Integrate" min=1.0 max=30.0 step=1.0
  out "APD Display Freq. (Hz)":dbl=6.666666666666667 caption="Freq. (Hz)"
  out "APD Display Period (s)":dbl=0.15 caption="Period (s)"
  out "FFT 1":cluster{"f0":dbl, "df":dbl, "magnitude":dbl[]}[](graph)=[{"f0"=0.0, "df"=3.3333333333333335, "magnitude"=array[10000 elements]}, {"f0"=0.0, "df"=3.3333333333333335, "magnitude"=array[10000 elements]}]
  out "FFT 2":cluster{"f0":dbl, "df":dbl, "magnitude":dbl[]}[](graph)
  in  "FFT 1 Choice 1":u16(ring) items=["T1 Y", "T1 X", "T1 Sum", "T2 Y", "T2 X", "T2 Sum", "T1 FB X", "T1 FB Sum", "T2 FB X", "T2 FB Sum", "PSD Y", "PSD X", "PSD Y Sum", "none"]
  in  "FFT 2 Choice 1":u16(ring)=13 items=["T1 Y", "T1 X", "T1 Sum", "T2 Y", "T2 X", "T2 Sum", "T1 FB X", "T1 FB Sum", "T2 FB X", "T2 FB Sum", "PSD Y", "PSD X", "PSD Y Sum", "none"]
  in  "FFT 1 Choice 2":u16(ring)=1 items=["T1 Y", "T1 X", "T1 Sum", "T2 Y", "T2 X", "T2 Sum", "T1 FB X", "T1 FB Sum", "T2 FB X", "T2 FB Sum", "PSD Y", "PSD X", "PSD Y Sum", "none"]
  in  "FFT 2 Choice 2":u16(ring)=13 items=["T1 Y", "T1 X", "T1 Sum", "T2 Y", "T2 X", "T2 Sum", "T1 FB X", "T1 FB Sum", "T2 FB X", "T2 FB Sum", "PSD Y", "PSD X", "PSD Y Sum", "none"]
  in  "Compute FFT":bool
  in  "Reset FFT":bool
  in  "# Spectra to Ave.":dbl=25.0
  out "Ave. Time (s)":dbl=7.5
  out "1 Channel":waveform(dbl)(graph)={"t0"=timestamp(0 s since 1904-01-01), "dt"=1.4999999999999999e-05, "Y"=array[20000 elements], "attributes"=variant("NI_ChannelName"=variant(string "T1 Y"))}
  out "Slow mean":dbl=-0.01200226252817839 format="%0.2f"
  in  "Slow mean N ave.":dbl=1.0 min=1.0 step=1.0
  out "Mean Intensity":dbl=-0.01200226252817839
  out "Sigma":dbl=0.006252248742901159
  out "Sigma/Mean":dbl=-0.5209225117532966
  in  "Subtract mean":bool
  in  "High Res. Display":u16(ring)=1 items=["T1 Y", "T1 X", "T1 Sum", "T2 Y", "T2 X", "T2 Sum", "T1 FB X", "T1 FB Sum", "T2 FB X", "T2 FB Sum", "PSD Y", "PSD X", "PSD Y Sum"]
  out "APD 1 Rate (Hz)":dbl=2627.0 format="%#_3p"
  in  "Tab Control":T5(tab)
  in  "11":bool
  out "Stage Moving":bool
  in  "Read Cal":bool
  in  "Confocal Linescan":bool
  in  "Speed (nm/s)":dbl=100.0
  in  "Furthest Withdraw (MHz)":dbl=15.0
  in  "Confocal Image":bool
  in  "Round T1 X":bool caption="Round"
  in  "T1 offset_x (mV)":dbl=93.7813251237406 format="%#_2g"
  in  "T1 kappa_x (pN/nm)":dbl=0.23595084426668553 min=0.0 step=0.001 format="%#_2g"
  out "Total Time (s)":dbl=60.0
  in  "Start Saving":bool
  in  "Cal sets to save":u32=25 min=1 step=1
  in  "Comment (data description)":string="testing confocal setup"
  out "Calibrating Trap...":bool
  in  "Trap 2 (ON/OFF)":bool
  in  "Trap 1 (ON/OFF)":bool
  in  "Save Calibration":bool
  in  "N sets to save":u32=200 caption="N Sets"
  in  "Save N Sets":bool
  out "Save file name":path=path "E:/Data/111017/111017_001.dat"
  in  "Save ave N":dbl=500.0 caption="Averaging Factor"
  out "Saving...":bool
  in  "Stop Saving":bool
  out "Progress":u16(slide) scale=0.0..100.0
  out "Manipulating Trap":bool
  out "Buffer Status":dbl(slide) scale=0.0..1.0
  out "Overflow (data lost)":bool
  in  "Reset":bool
  out "Data Rate (Hz)":dbl=66666.66666666667 caption="Trap Data Rate (Hz)" format="%#_3p"
  out "Data Period (s)":dbl=1.4999999999999999e-05 caption="Trap Data Period (s)" format="%#_6p"
  out "Save Data Rate (Hz)":dbl=133.33333333333334 caption="Rate (Hz)" format="%#_6p"
  out "Save Data Period (s)":dbl=0.0075 caption="Period (s)" format="%#_6p"
  in  "T1 alpha_x (nm/V)":dbl=756.882362133965 step=10.0 format="%#_3g"
  in  "T2 alpha_x (nm/V)":dbl=622.8162591967915 step=10.0 format="%#_3g"
  in  "T2 kappa_x (pN/nm)":dbl=0.2575992919520022 min=0.0 step=0.001 format="%#_2g"
  in  "T2 offset_x (mV)":dbl=85.47545600324118 format="%#_2g"
  in  "BD 1 Frequency 1 (MHz)":dbl=69.75 caption="T1 X (MHz)" min=60.0 max=90.0 step=1.0 format="%#_6p"
  in  "BD 1 Frequency 2 (MHz)":dbl=85.0 caption="T2 X (MHz)" min=60.0 max=90.0 step=1.0 format="%#_6p"
  in  "Green Laser ON/Interlacing":bool=TRUE
  in  "Round T2 X":bool caption="Round"
  in  "AO1":dbl(slide)=7.2279940183721445 caption="Confocal Y (V)" min=0.0 max=10.0 step=0.01 scale=0.0..10.0 scale format="%_1f"
  in  "AO2":dbl(slide)=1.225451826532792 caption="Confocal X (V)" min=0.0 max=10.0 step=0.01 scale=0.0..10.0 scale format="%_1f"
  in  "Trap Raster Scan":bool
  out "Raster Scanning...":bool
  in  "Trap Delta (MHz)":dbl=15.25
  in  "Setpoints (V)":cluster{"Set 1":dbl, "Set 2":dbl}={"Set 1"=9.0, "Set 2"=9.0}
  in  "Green FB Setpoint (mV)":dbl=90.0
  in  "Fish for Tether":bool
  in  "Position Label 5":string="upper flow spot (UvrD)" caption="5"
  in  "Move to Position":bool
  in  "Position":dbl=1.0 min=1.0 max=10.0 step=1.0
  in  "Set Position":bool
  in  "Saved Stage Positions":dbl[][](array[numeric])=[[1.0, 0.0, 0.0, 0.0], [2.0, -0.63535, -2.1332, -0.02485], [3.0, 1.5, -0.5, 0.0], [4.0, -0.03433, -2.49081, -0.0084], [5.0, 1.5, -2.0, -0.015], [6.0, 0.0, 0.0, 0.0], [7.0, 0.0, 0.0, 0.0], [8.0, 0.0, 0.0, 0.0], [9.0, 0.0, 0.0, 0.0], [10.0, 0.0, 0.0, 0.0]]
  in  "Move to Position 5":bool
  in  "z nudge increment (um)":dbl=0.5
  in  "+z":bool
  in  "Position 1 Label":string="Lower capillary (DNA beads)" caption="1"
  in  "Set Position 1":bool
  in  "Set Position 2":bool
  in  "Set Position 3":bool
  in  "Set Position 4":bool
  in  "Move to Position 3":bool
  in  "Move to Position 4":bool
  in  "Move to Position 2":bool
  in  "Move to Position 1":bool
  in  "Position 2 Label":string="Upper capillary (ADig beads)" caption="2"
  in  "Position 3 Label":string="lower flow spot (ATP)" caption="3"
  in  "Position 4 Label":string="Dump beads" caption="4"
  in  "-z":bool
  in  "Set Position 5":bool
  out "Stage Control Serial Error":errorcluster
  in  "Read Harvard":bool
  in  "Clear Volume":bool caption="Clear Infused Volume"
  in  "Flow rate (uL/h)":dbl=100.0
  in  "Flush rate (uL/m)":dbl=100.0
  in  "Flush Sample":bool
  in  "Volume (uL)":dbl=100.0
  out "read buffer":string
  out "Serial Settings:Number of Bytes at Serial Port":u32
  in  "write buffer":string
  in  "Tab Control 2":T6(tab)=enum."Feedback on Trap Position"
  out "Total Counts (ticks)":u32=600
  in  "Trap ON/OFF X or Y Amp?":bool=TRUE
  in  "Oscillate Set 1":bool
  in  "Trap 1 ON":bool
  in  "Number Interlace Sets":u8=3 min=1 max=3
  in  "DIO count 3 (ticks)":u32=200
  in  "DIO count 2 (ticks)":u32=200
  in  "DIO count 1 (ticks)":u32=200
  in  "BD 2 Amplitude 3 (%)":dbl min=0.0 max=50.0 step=1.0
  in  "BD 2 Amplitude 2 (%)":dbl min=0.0 max=50.0 step=1.0
  in  "BD 2 Amplitude 1 (%)":dbl min=0.0 max=50.0 step=1.0
  in  "BD 1 Amplitude 3 (%)":dbl min=0.0 max=50.0 step=1.0
  in  "BD 1 Amplitude 2 (%)":dbl=35.0 min=0.0 max=50.0 step=1.0
  in  "BD 1 Amplitude 1 (%)":dbl=10.0 min=0.0 max=50.0 step=1.0
  in  "BD 2 Frequency 3 (MHz)":dbl=26.0 min=0.0 max=40.0 step=1.0 format="%#_6p"
  in  "BD 1 Frequency 3 (MHz)":dbl=70.0 min=60.0 max=90.0 step=1.0 format="%#_6p"
  in  "BD 2 Frequency 2 (MHz)":dbl=26.0 min=0.0 max=40.0 step=1.0 format="%#_6p"
  in  "BD 2 Frequency 1 (MHz)":dbl=26.0 min=0.0 max=40.0 step=1.0 format="%#_6p"
  in  "Not-Interlacing Set":enum32{"Set 1", "Set 2", "Set 3"}(radio)
  in  "Interlace":bool=TRUE
  in  "Trap 2 ON":bool
  in  "Trap 3 ON":bool
  in  "Scan axis 2":bool=TRUE
  in  "Osc. freq. (Hz)":dbl=0.25
  in  "Osc. amp. (MHz)":dbl=2.0
  out "Coords":T7
  in  "Manipulation Scaling":cluster{"Horizontal":dbl, "Vertical":dbl}={"Horizontal"=0.075, "Vertical"=0.01}
  in  "Freq or Amp switch first":bool=TRUE
  in  "Swap F1 and F2":bool
  in  "Freq switch delay":u16
  in  "Amp switch delay":u16=5
  in  "MCL Step Increment (V_int)":dbl=3.0
  out "Time to Finish All (min)":dbl=0.13986 format="%#_2p"
  in  "Scan Speed (nm/s)":dbl=100.0
  in  "Scan Range (nm)":dbl=420.0
  in  "Step Size (nm)":dbl=1.0
  in  "MCL/AOM Scale Tweak":dbl=1.0
  in  "MCL Step Position Ratio":dbl=0.5
  in  "Move MCL Also?":bool=TRUE
  out "Final sep (nm)":dbl=1470.750000000001
  out "Initial sep (nm)":dbl=1050.75
  out "Save index":dbl=1.0
  out "Final delta (MHz)":dbl=18.66463414634147
  out "Initial delta (MHz)":dbl=15.25
  out "Final freq. (MHz)":dbl=66.33536585365853
  out "Initial freq. (MHz)":dbl=69.75
  in  "Saved AOD Raster Scan Parameter Sets":T8(array[cluster])=[{"Scan Range AOD (nm) 2"=500.0, "Step Size AOD (nm) 2"=1.0, "Scan Speed AOD (nm/s) 2"=100.0, "Number of scans (AOD) 2"=1, "Label"="offset curve"}, {"Scan Range AOD (nm) 2"=420.0, "Step Size AOD (nm) 2"=1.0, "Scan Speed AOD (nm/s) 2"=100.0, "Number of scans (AOD) 2"=1, "Label"="hp raster check"}, {"Scan Range AOD (nm) 2"=6.8, "Step Size AOD (nm) 2"=0.34, "Scan Speed AOD (nm/s) 2"=0.34, "Number of scans (AOD) 2"=1, "Label"="3.4 kbp - 1 bp steps"}, {"Scan Range AOD (nm) 2"=215.0, "Step Size AOD (nm) 2"=1.0, "Scan Speed AOD (nm/s) 2"=100.0, "Number of scans (AOD) 2"=3, "Label"="dt14 1 14 MHz start"}, {"Scan Range AOD (nm) 2"=450.0, "Step Size AOD (nm) 2"=1.0, "Scan Speed AOD (nm/s) 2"=100.0, "Number of scans (AOD) 2"=1, "Label"="dt14 2 small beads"}]
  in  "Load parameters":bool
  out "Scan Range (MHz)":dbl=-3.4146341463414633
  in  "Restart DMA? (AOD)":bool=TRUE caption="Restart DMA?"
  out "Incr. int (AOD)":i64=-7759651845
  out "Time/Scan (s) (AOD)":dbl=4.1958 format="%#_2p"
  out "Data points/scans":dbl=559440.0
  out "Data points/scan (f/b)":dbl=559440.0
  in  "Save scans":bool=TRUE
  out "AOD Scan I":u64 caption="Scan I"
  in  "Continuous AOD Scanning":bool caption="Continuous Scanning"
  in  "Abort AOD Scan":bool caption="Abort Scan"
  in  "Scan BD":bool=TRUE
  out "Cycles/step (AOD)":u64=666 format="%.3p"
  in  "Number of F/B Scans (AOD)":u16=1 min=1
  out "Scan steps (AOD)":u64=420
  out "Scan Increment (MHz)":dbl=-0.008149484836137144
  out "AOD Scanning":bool caption="Scanning"
  in  "Start AOD Scan":bool caption="Start Scan"
  out "N sets should be saved":dbl=27.972
  out "Progress 2":u16(slide) caption="Progress" scale=0.0..100.0
  in  "Abort save 2":bool caption="Abort save"
  in  "Trap 1 Bead Size (nm)":dbl=860.0
  in  "Trap 2 Bead Size (nm)":dbl=790.0
  out "MCL Count":dbl=782931.6080202643
  in  "All FB On/Off":bool=TRUE
